vi "InitWaveform.vi"(11 "Refnum in":refnum<k21>) -> (3 "Waveform":waveform(dbl))   [LabVIEW 2018]
uses:
  <resource>/objmgr/daqmx.rc
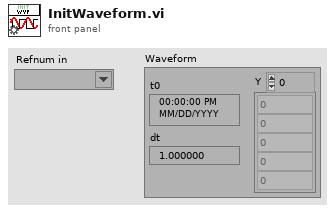
[diagram p1: front panel]
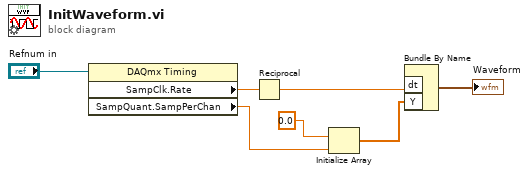
[diagram p0: block diagram]
diagram:
  n1 = property class="DAQmx Timing"(reference="Refnum in") -> ("SampClk.Rate"=w2:dbl, "SampQuant.SampPerChan"=w1:dbl)  [unwired: 1 in, 2 out]
  n2 = Reciprocal(x=w2) -> (1/x=w3:dbl)
  n3 = Initialize Array(0.0 ("element"), w1) -> (w6:dbl[])
  n4 = Bundle By Name("dt"=w3, "Y"=w6) -> (→"Waveform":waveform(dbl))  [unwired: 1 in]
